vi "Tell Child.vi"(4 "Priority":bool, 6 "UID":string, 7 "Actor in":refnum<class "Actor.lvclass">, 9 "Error":errorcluster, 10 "Actor":refnum<class "Actor.lvclass">) -> (0 "Error out":errorcluster)   [LabVIEW 2025, in "jettl.lvlib" / "Stopped Msg.lvlib"]
uses:
  Stopped Msg.lvlib
  Actor/Actor/Actor.lvclass
  Stopped Msg/Stopped Msg.lvclass
  C:/git/jettl/src/jettl/jettl/Msg/Msg.lvclass
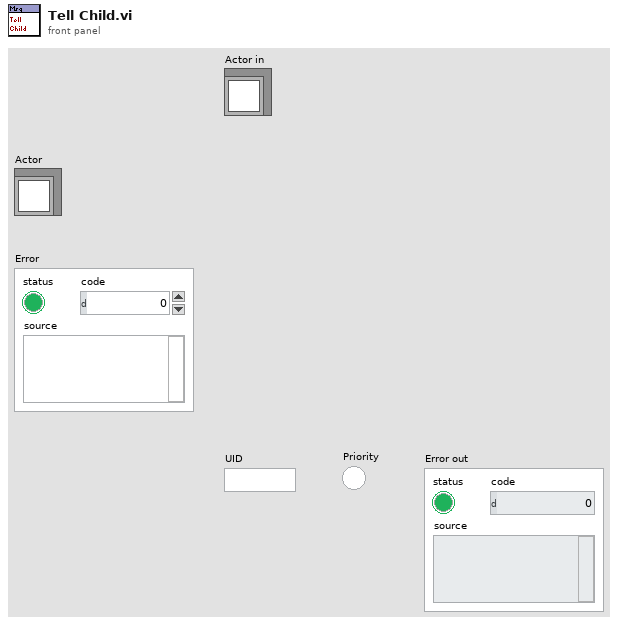
[diagram p1: front panel]
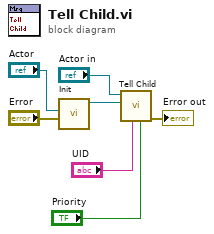
[diagram p0: block diagram]
diagram:
  n1 = call "Init.vi"("Error"="Error", "Actor"="Actor") -> ("Stopped Msg out"=w3:refnum<class "Stopped Msg.lvclass">)  [unwired: 9 in]
  n2 = call-dynamic "Tell Child.vi"("Priority"="Priority", "UID"="UID", "Msg"=w3, "Actor in"="Actor in") -> ("Error out"=→"Error out":errorcluster)  [unwired: 7 in]
